vi "Read VISA resource name.vi"(11 "Instrument in":refnum<class "Instrument.lvclass">) -> (2 "VISA resource name":refnum<visa-resource-name>, 3 "Instrument out":refnum<class "Instrument.lvclass">)   [LabVIEW 2020, in "Instrument.lvclass"]
uses:
  Instrument.lvclass
  Instrument.lvclass/Instrument.ctl
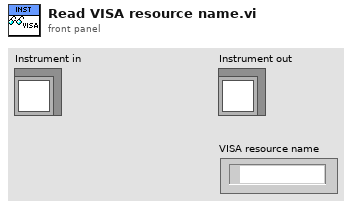
[diagram p1: front panel]
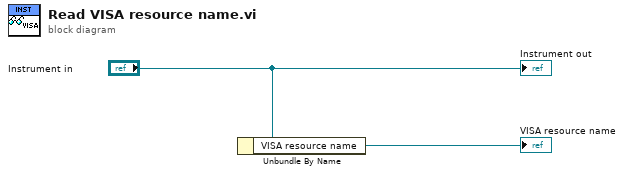
[diagram p0: block diagram]
diagram:
  n1 = Unbundle By Name("Instrument in") -> ("VISA resource name"=→"VISA resource name":refnum<visa-resource-name>)
  "Instrument out" <- "Instrument in"
